vi "Trash pathname files.vi"(0 "Pass through variable.":i32) -> (1 "Pass through variable.":i32, 2 "Error bundle out.":errorcluster)   [LabVIEW 2010]
panel:
  in  "Case Constant\n(See Context Help)":bool=TRUE
  # "Input:"
  # "Output:"
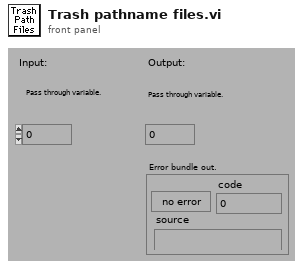
[diagram p1: front panel]
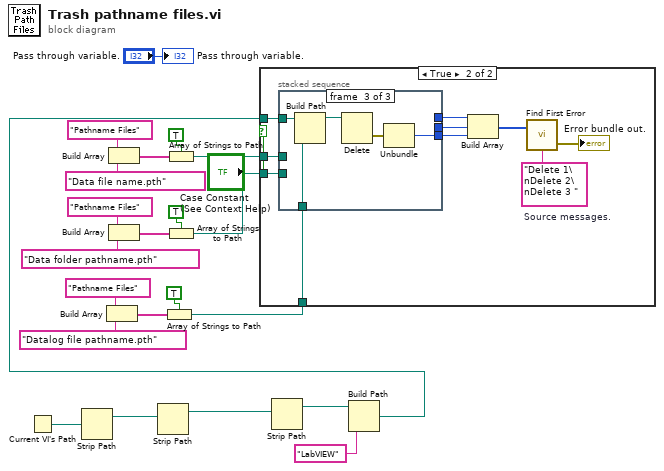
[diagram p0: block diagram]
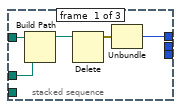
[diagram p3: hidden frame]
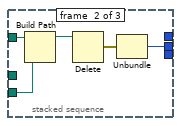
[diagram p4: hidden frame]
diagram:
  n1 = Current VI's Path() -> (path=w6:path)
  n2 = Strip Path(path=w6) -> (stripped path=w5:path)  [unwired: 1 out]
  n3 = Build Array("Pathname Files", "Datalog file pathname.pth") -> (w15:string[])
  n4 = Build Array("Pathname Files", "Data file name.pth") -> (w23:string[])
  n5 = Build Array("Pathname Files", "Data folder pathname.pth") -> (w19:string[])
  n6 = Strip Path(path=w5) -> (stripped path=w4:path)  [unwired: 1 out]
  n7 = Array of Strings to Path(0:w15, 1:TRUE) -> (2:w9:path)
  n8 = Array of Strings to Path(0:w23, 1:TRUE) -> (2:w8:path)
  n9 = Array of Strings to Path(0:w19, 1:TRUE) -> (2:w11:path)
  n10 = Strip Path(path=w4) -> (stripped path=w3:path)  [unwired: 1 out]
  n11 = Build Path(base path=w3, name or relative path="LabVIEW") -> (appended path=w1:path)
  n12 = case shown="True" "Case Constant\n(See Context Help)" {
    tunnel: w1 -> [_ w33]
    tunnel: w8 -> [_ w32]
    tunnel: w11 -> [_ w31]
    tunnel: w9 -> [_ w30]
    frame False {
    }
    frame True {
      w26 = "Delete 1\nDelete 2\nDelete 3 "  # Source messages.
      n13 = stacked-sequence {
        tunnel: w33 -> [w37 w41 w48]
        tunnel: w32 -> [w38 _ _]
        tunnel: w31 -> [_ w43 _]
        tunnel: w30 -> [_ _ w47]
        tunnel: [w34 _ _] -> w29
        tunnel: [_ w39 _] -> w28
        tunnel: [_ _ w44] -> w27
        frame #0 {
          n14 = Build Path(base path=w37, name or relative path=w38) -> (appended path=w35:path)
          n15 = Delete(path (use dialog)=w35) -> (error out=w36:errorcluster)  [unwired: 1 in, 5 out]
          n16 = Unbundle(w36) -> ("code"=w34:i32)  [unwired: 2 out]
        }
        frame #1 {
          n17 = Build Path(base path=w41, name or relative path=w43) -> (appended path=w42:path)
          n18 = Delete(path (use dialog)=w42) -> (error out=w40:errorcluster)  [unwired: 1 in, 5 out]
          n19 = Unbundle(w40) -> ("code"=w39:i32)  [unwired: 2 out]
        }
        frame #2 {
          n20 = Build Path(base path=w48, name or relative path=w47) -> (appended path=w46:path)
          n21 = Delete(path (use dialog)=w46) -> (error out=w45:errorcluster)  [unwired: 1 in, 5 out]
          n22 = Unbundle(w45) -> ("code"=w44:i32)  [unwired: 2 out]
        }
      }
      n23 = Build Array(w29, w28, w27) -> (w25:i32[])
      n24 = call <vilib>:"Find First Error.vi"("source messages"=w26, "error codes"=w25) -> ("error out"=→"Error bundle out.":errorcluster)  [unwired: 1 in, 2 out]
    }
  }
  "Pass through variable." <- "Pass through variable."
